vi "lab4_3.vi"() -> ()   [LabVIEW 2021]
panel:
  out "X-Y":dbl
  out "X+Y":dbl
  in  "Y":dbl
  in  "X":dbl
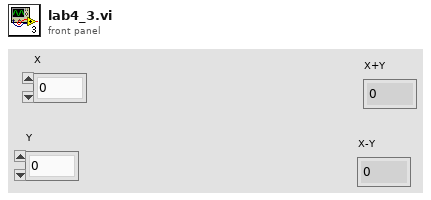
[diagram p1: front panel]
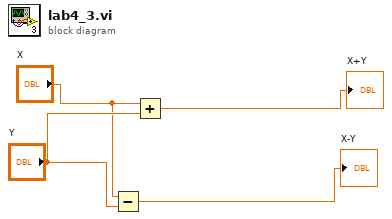
[diagram p0: block diagram]
diagram:
  n1 = Subtract(x="X", y="Y") -> (x-y=→"X-Y":dbl)
  n2 = Add(x="X", y="Y") -> (x+y=→"X+Y":dbl)
